vi "myRIO_BRig_RT__Case_Exp_subState_LC__initTrial__v4.vi"(0 "input_dataCurrent":u16[](array[numeric]), 1 "input_dataExp":u16[](array[numeric]), 2 "input_dataLC":u16[](array[numeric]), 6 "input_spout":enum16{"Left", "Right"}(ring), 8 "input_dataTrial":u16[][](array[numeric])) -> (10 "output_dataTrial":u16[][](array[numeric]), 11 "output_LR_Wrong_Laser_l2":bool, 12 "output_dataCurrent":u16[](array[numeric]), 13 "output_LR_Reward_Laser_l2":bool, 14 "output_LR_Reward_Event_l1":bool, 15 "output_LR_Wrong_Event_l1":bool, 16 "output_LR_Reward_Laser_l1":bool, 17 "output_LR_Wrong_Laser_l1":bool, 18 "output_LR_Reward_Event_l2":bool, 19 "output_LR_Wrong_Event_l2":bool)   [LabVIEW 2014]
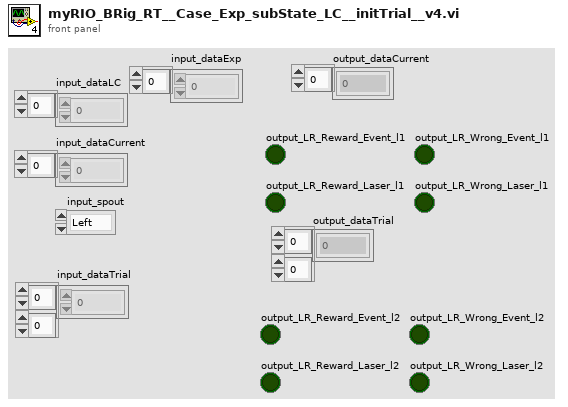
[diagram p1: front panel]
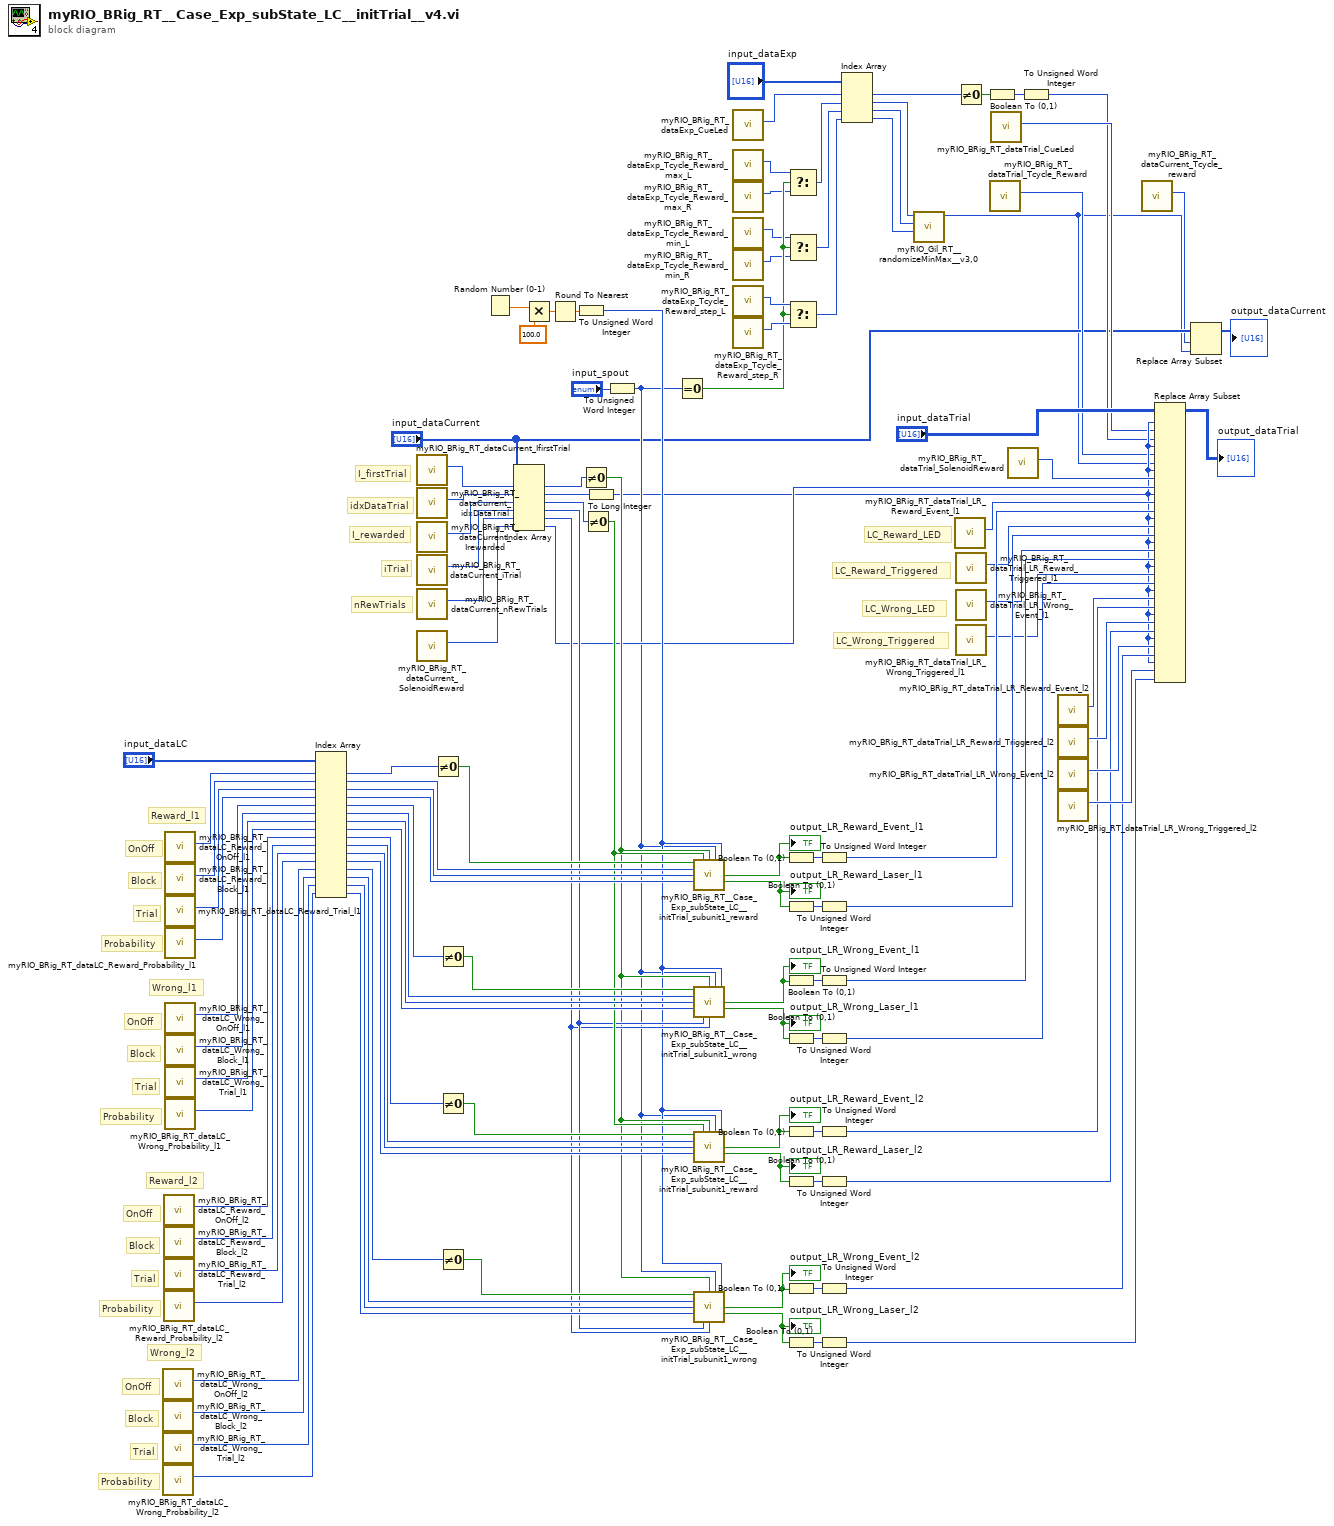
[diagram p0: block diagram]
diagram:
  # "Probability"
  # "Trial"
  # "Block"
  # "OnOff"
  # "Wrong_l2"
  # "Reward_l2"
  # "Probability"
  # "Trial"
  # "Block"
  # "OnOff"
  # "nRewTrials"
  # "iTrial"
  # "I_rewarded"
  # "LC_Wrong_Triggered"
  # "LC_Wrong_LED"
  # "LC_Reward_Triggered"
  # "LC_Reward_LED"
  # "idxDataTrial"
  # "Probability"
  # "Trial"
  # "Block"
  # "OnOff"
  # "Wrong_l1"
  # "I_firstTrial"
  # "Reward_l1"
  # "Probability"
  # "Trial"
  # "Block"
  # "OnOff"
  n1 = call "myRIO_BRig_RT_dataLC_Wrong_OnOff_l2.vi"() -> ("output_Wrong_OnOff_l2"=w76:i32)  [unwired: 11 in]
  n2 = call "myRIO_BRig_RT_dataLC_Wrong_Block_l2.vi"() -> ("output_Wrong_Block_l2"=w75:i32)  [unwired: 11 in]
  n3 = call "myRIO_BRig_RT_dataLC_Wrong_Trial_l2.vi"() -> ("output_Wrong_Trial_l2"=w74:i32)  [unwired: 11 in]
  n4 = call "myRIO_BRig_RT_dataLC_Wrong_Probability_l2.vi"() -> ("output_Wrong_Probability_l2"=w73:i32)  [unwired: 11 in]
  n5 = call "myRIO_BRig_RT_dataLC_Reward_OnOff_l2.vi"() -> ("output_Reward_OnOff_l2"=w80:i32)  [unwired: 11 in]
  n6 = call "myRIO_BRig_RT_dataLC_Reward_Block_l2.vi"() -> ("output_Reward_Block_l2"=w79:i32)  [unwired: 11 in]
  n7 = call "myRIO_BRig_RT_dataLC_Reward_Trial_l2.vi"() -> ("output_Reward_Trial_l2"=w78:i32)  [unwired: 11 in]
  n8 = call "myRIO_BRig_RT_dataLC_Reward_Probability_l2.vi"() -> ("output_Reward_Probability_l2"=w77:i32)  [unwired: 11 in]
  n9 = call "myRIO_BRig_RT_dataLC_Reward_OnOff_l1.vi"() -> ("output_Reward_OnOff_l1"=w118:i32)  [unwired: 11 in]
  n10 = call "myRIO_BRig_RT_dataLC_Reward_Block_l1.vi"() -> ("output_Reward_Block_l1"=w117:i32)  [unwired: 11 in]
  n11 = call "myRIO_BRig_RT_dataLC_Reward_Trial_l1.vi"() -> ("output_Reward_Trial_l1"=w116:i32)  [unwired: 11 in]
  n12 = call "myRIO_BRig_RT_dataLC_Reward_Probability_l1.vi"() -> ("output_Reward_Probability_l1"=w115:i32)  [unwired: 11 in]
  n13 = call "myRIO_BRig_RT_dataLC_Wrong_OnOff_l1.vi"() -> ("output_Wrong_OnOff_l1"=w108:i32)  [unwired: 11 in]
  n14 = call "myRIO_BRig_RT_dataLC_Wrong_Block_l1.vi"() -> ("output_Wrong_Block_l1"=w109:i32)  [unwired: 11 in]
  n15 = call "myRIO_BRig_RT_dataLC_Wrong_Trial_l1.vi"() -> ("output_Wrong_Trial_l1"=w110:i32)  [unwired: 11 in]
  n16 = call "myRIO_BRig_RT_dataLC_Wrong_Probability_l1.vi"() -> ("output_Wrong_Probability_l1"=w111:i32)  [unwired: 11 in]
  n17 = Index Array(array="input_dataLC", index #1=w118, index #2=w117, index #3=w116, index #4=w115, index #5=w108, index #6=w109, index #7=w110, index #8=w111, index #9=w80, index #10=w79, index #11=w78, index #12=w77, index #13=w76, index #14=w75, index #15=w74, index #16=w73) -> (element #1=w114:u16, element #2=w65:u16, element #3=w64:u16, element #4=w63:u16, element #5=w106:u16, element #6=w59:u16, element #7=w58:u16, element #8=w57:u16, element #9=w68:u16, element #10=w53:u16, element #11=w52:u16, element #12=w51:u16, element #13=w67:u16, element #14=w46:u16, element #15=w45:u16, element #16=w44:u16)
  n18 = call "myRIO_BRig_RT_dataCurrent_IfirstTrial.vi"() -> ("output_I_firstTrial"=w113:i32)  [unwired: 11 in]
  n19 = call "myRIO_BRig_RT_dataCurrent_idxDataTrial.vi"() -> ("output_idxDataTrial"=w105:i32)  [unwired: 11 in]
  n20 = call "myRIO_BRig_RT_dataCurrent_Irewarded.vi"() -> ("output_I_rewarded"=w89:i32)  [unwired: 11 in]
  n21 = call "myRIO_BRig_RT_dataCurrent_iTrial.vi"() -> ("output_iTrial"=w87:i32)  [unwired: 11 in]
  n22 = call "myRIO_BRig_RT_dataCurrent_nRewTrials.vi"() -> ("output_nRewTrials"=w86:i32)  [unwired: 11 in]
  n23 = call "myRIO_BRig_RT_dataCurrent_SolenoidReward.vi"() -> ("output_SolenoidReward"=w85:i32)  [unwired: 11 in]
  n24 = Not Equal To 0?(x=w114) -> (x != 0?=w66:bool)
  n25 = Not Equal To 0?(x=w106) -> (x != 0?=w60:bool)
  n26 = Not Equal To 0?(x=w68) -> (x != 0?=w54:bool)
  n27 = Not Equal To 0?(x=w67) -> (x != 0?=w47:bool)
  n28 = Random Number (0-1)() -> (number: 0 to 1=w81:dbl)
  n29 = Index Array(array="input_dataCurrent", index #1=w113, index #2=w105, index #3=w89, index #4=w87, index #5=w86, index #6=w85) -> (element #1=w112:u16, element #2=w104:u16, element #3=w88:u16, element #4=w43:u16, element #5=w42:u16, element #6=w37:u16)
  n30 = Multiply(x=w81, y=100.0) -> (x*y=w82:dbl)
  n31 = Round To Nearest(number=w82) -> (nearest integer value=w83:dbl)
  n32 = To Unsigned Word Integer(number=w83) -> (unsigned 16bit integer=w40:u16)
  n33 = Not Equal To 0?(x=w112) -> (x != 0?=w41:bool)
  n34 = Not Equal To 0?(x=w88) -> (x != 0?=w50:bool)
  n35 = To Long Integer(number=w104) -> (32bit integer=w8:i32)
  n36 = To Unsigned Word Integer(number="input_spout") -> (unsigned 16bit integer=w22:u16)
  n37 = Equal To 0?(x=w22) -> (x = 0?=w19:bool)
  n38 = call "myRIO_BRig_RT__Case_Exp_subState_LC__initTrial_subunit1_reward.vi"("input_LR_OnOff"=w66, "input_I_rewarded"=w50, "input_I_firstTrial"=w41, "input_spout"=w22, "input_randomNumber"=w40, "input_LR_Block"=w65, "input_LR_Trial"=w64, "input_LR_Probability"=w63) -> ("output_LR_Event"=w62:bool, "output_LR_Laser"=w61:bool)  [unwired: 6 in]
  "output_LR_Reward_Laser_l1" <- w61
  "output_LR_Reward_Event_l1" <- w62
  n39 = call "myRIO_BRig_RT__Case_Exp_subState_LC__initTrial_subunit1_wrong.vi"("input_LR_OnOff"=w60, "input_I_firstTrial"=w41, "input_spout"=w22, "input_randomNumber"=w40, "input_LR_Block"=w59, "input_LR_Trial"=w58, "input_LR_Probability"=w57, "input_iTrial"=w43, "input_nRewTrials"=w42) -> ("output_LR_Event"=w56:bool, "output_LR_Laser"=w55:bool)  [unwired: 5 in]
  "output_LR_Wrong_Laser_l1" <- w55
  "output_LR_Wrong_Event_l1" <- w56
  n40 = call "myRIO_BRig_RT__Case_Exp_subState_LC__initTrial_subunit1_reward.vi"("input_LR_OnOff"=w54, "input_I_rewarded"=w50, "input_I_firstTrial"=w41, "input_spout"=w22, "input_randomNumber"=w40, "input_LR_Block"=w53, "input_LR_Trial"=w52, "input_LR_Probability"=w51) -> ("output_LR_Event"=w49:bool, "output_LR_Laser"=w48:bool)  [unwired: 6 in]
  "output_LR_Reward_Laser_l2" <- w48
  "output_LR_Reward_Event_l2" <- w49
  n41 = call "myRIO_BRig_RT__Case_Exp_subState_LC__initTrial_subunit1_wrong.vi"("input_LR_OnOff"=w47, "input_I_firstTrial"=w41, "input_spout"=w22, "input_randomNumber"=w40, "input_LR_Block"=w46, "input_LR_Trial"=w45, "input_LR_Probability"=w44, "input_iTrial"=w43, "input_nRewTrials"=w42) -> ("output_LR_Event"=w39:bool, "output_LR_Laser"=w38:bool)  [unwired: 5 in]
  "output_LR_Wrong_Laser_l2" <- w38
  "output_LR_Wrong_Event_l2" <- w39
  n42 = call "myRIO_BRig_RT_dataExp_CueLed.vi"() -> ("output_CueLed"=w27:i32)  [unwired: 11 in]
  n43 = call "myRIO_BRig_RT_dataExp_Tcycle_Reward_max_L.vi"() -> ("output_Tcycle_Reward_max_L"=w15:i32)  [unwired: 11 in]
  n44 = call "myRIO_BRig_RT_dataExp_Tcycle_Reward_max_R.vi"() -> ("output_Tcycle_Reward_max_R"=w16:i32)  [unwired: 11 in]
  n45 = call "myRIO_BRig_RT_dataExp_Tcycle_Reward_min_L.vi"() -> ("output_Tcycle_Reward_min_L"=w17:i32)  [unwired: 11 in]
  n46 = call "myRIO_BRig_RT_dataExp_Tcycle_Reward_min_R.vi"() -> ("output_Tcycle_Reward_min_R"=w18:i32)  [unwired: 11 in]
  n47 = call "myRIO_BRig_RT_dataExp_Tcycle_Reward_step_L.vi"() -> ("output_Tcycle_Reward_step_L"=w20:i32)  [unwired: 11 in]
  n48 = call "myRIO_BRig_RT_dataExp_Tcycle_Reward_step_R.vi"() -> ("output_Tcycle_Reward_step_R"=w21:i32)  [unwired: 11 in]
  n49 = Boolean To (0,1)(Boolean=w62) -> (0, 1=w100:i16)
  n50 = Boolean To (0,1)(Boolean=w61) -> (0, 1=w98:i16)
  n51 = Boolean To (0,1)(Boolean=w56) -> (0, 1=w94:i16)
  n52 = Boolean To (0,1)(Boolean=w55) -> (0, 1=w91:i16)
  n53 = Boolean To (0,1)(Boolean=w49) -> (0, 1=w72:i16)
  n54 = Boolean To (0,1)(Boolean=w48) -> (0, 1=w71:i16)
  n55 = Boolean To (0,1)(Boolean=w39) -> (0, 1=w70:i16)
  n56 = Boolean To (0,1)(Boolean=w38) -> (0, 1=w69:i16)
  n57 = Select(t=w15, s=w19, f=w16) -> (s? t:f=w14:i32)
  n58 = Select(t=w17, s=w19, f=w18) -> (s? t:f=w13:i32)
  n59 = Select(t=w20, s=w19, f=w21) -> (s? t:f=w12:i32)
  n60 = To Unsigned Word Integer(number=w100) -> (unsigned 16bit integer=w99:u16)
  n61 = To Unsigned Word Integer(number=w98) -> (unsigned 16bit integer=w96:u16)
  n62 = To Unsigned Word Integer(number=w94) -> (unsigned 16bit integer=w93:u16)
  n63 = To Unsigned Word Integer(number=w91) -> (unsigned 16bit integer=w90:u16)
  n64 = To Unsigned Word Integer(number=w72) -> (unsigned 16bit integer=w32:u16)
  n65 = To Unsigned Word Integer(number=w71) -> (unsigned 16bit integer=w31:u16)
  n66 = To Unsigned Word Integer(number=w70) -> (unsigned 16bit integer=w30:u16)
  n67 = To Unsigned Word Integer(number=w69) -> (unsigned 16bit integer=w29:u16)
  n68 = Index Array(array="input_dataExp", index #1=w27, index #2=w14, index #3=w13, index #4=w12) -> (element #1=w26:u16, element #2=w11:u16, element #3=w10:u16, element #4=w9:u16)
  n69 = call "myRIO_Gil_RT__randomizeMinMax__v3,0.vi"("Input_Increment"=w9, "Input_Min"=w10, "Input_Max"=w11) -> ("Output"=w2:u16)  [unwired: 8 in]
  n70 = call "myRIO_BRig_RT_dataTrial_LR_Reward_Event_l1.vi"() -> ("output_LR_Reward_Event_l1"=w101:i32)  [unwired: 11 in]
  n71 = Not Equal To 0?(x=w26) -> (x != 0?=w25:bool)
  n72 = call "myRIO_BRig_RT_dataTrial_LR_Reward_Triggered_l1.vi"() -> ("output_LR_Reward_Triggered_l1"=w97:i32)  [unwired: 11 in]
  n73 = call "myRIO_BRig_RT_dataTrial_LR_Wrong_Event_l1.vi"() -> ("output_LR_Wrong_Event_l1"=w95:i32)  [unwired: 11 in]
  n74 = call "myRIO_BRig_RT_dataTrial_LR_Wrong_Triggered_l1.vi"() -> ("output_LR_Wrong_Triggered_l1"=w92:i32)  [unwired: 11 in]
  n75 = Boolean To (0,1)(Boolean=w25) -> (0, 1=w24:i16)
  n76 = call "myRIO_BRig_RT_dataTrial_Tcycle_Reward.vi"() -> ("output_Tcycle_Reward"=w5:i32)  [unwired: 11 in]
  n77 = call "myRIO_BRig_RT_dataTrial_CueLed.vi"() -> ("output_CueLed"=w7:i32)  [unwired: 11 in]
  n78 = call "myRIO_BRig_RT_dataTrial_SolenoidReward.vi"() -> ("output_SolenoidReward"=w23:i32)  [unwired: 11 in]
  n79 = To Unsigned Word Integer(number=w24) -> (unsigned 16bit integer=w6:u16)
  n80 = call "myRIO_BRig_RT_dataTrial_LR_Reward_Event_l2.vi"() -> ("output_LR_Reward_Event_l2"=w36:i32)  [unwired: 11 in]
  n81 = call "myRIO_BRig_RT_dataTrial_LR_Reward_Triggered_l2.vi"() -> ("output_LR_Reward_Triggered_l2"=w35:i32)  [unwired: 11 in]
  n82 = call "myRIO_BRig_RT_dataTrial_LR_Wrong_Event_l2.vi"() -> ("output_LR_Wrong_Event_l2"=w34:i32)  [unwired: 11 in]
  n83 = call "myRIO_BRig_RT_dataTrial_LR_Wrong_Triggered_l2.vi"() -> ("output_LR_Wrong_Triggered_l2"=w33:i32)  [unwired: 11 in]
  n84 = call "myRIO_BRig_RT_dataCurrent_Tcycle_reward.vi"() -> ("output_Tcycle_reward"=w3:i32)  [unwired: 11 in]
  n85 = Replace Array Subset(array="input_dataTrial", new element #1=w6, index (row) #1=w8, index (col) #1=w7, new element #2=w2, index (row) #2=w8, index (col) #2=w5, new element #3=w37, index (row) #3=w8, index (col) #3=w23, new element #4=w99, index (row) #4=w8, index (col) #4=w101, new element #5=w96, index (row) #5=w8, index (col) #5=w97, new element #6=w93, index (row) #6=w8, index (col) #6=w95, new element #7=w90, index (row) #7=w8, index (col) #7=w92, new element #8=w32, index (row) #8=w8, index (col) #8=w36, new element #9=w31, index (row) #9=w8, index (col) #9=w35, new element #10=w30, index (row) #10=w8, index (col) #10=w34, new element #11=w29, index (row) #11=w8, index (col) #11=w33) -> (→"output_dataTrial":u16[][])
  n86 = Replace Array Subset(array="input_dataCurrent", new element=w2, index=w3) -> (→"output_dataCurrent":u16[])
